vi "DeleteSearch.vi"(10 "EventQueue":T2(array[cluster]), 11 "Event":T3) -> (2 "Found":bool, 3 "Index":i32)   [LabVIEW 2014]
uses:
  TypeDefs/Point2D.ctl
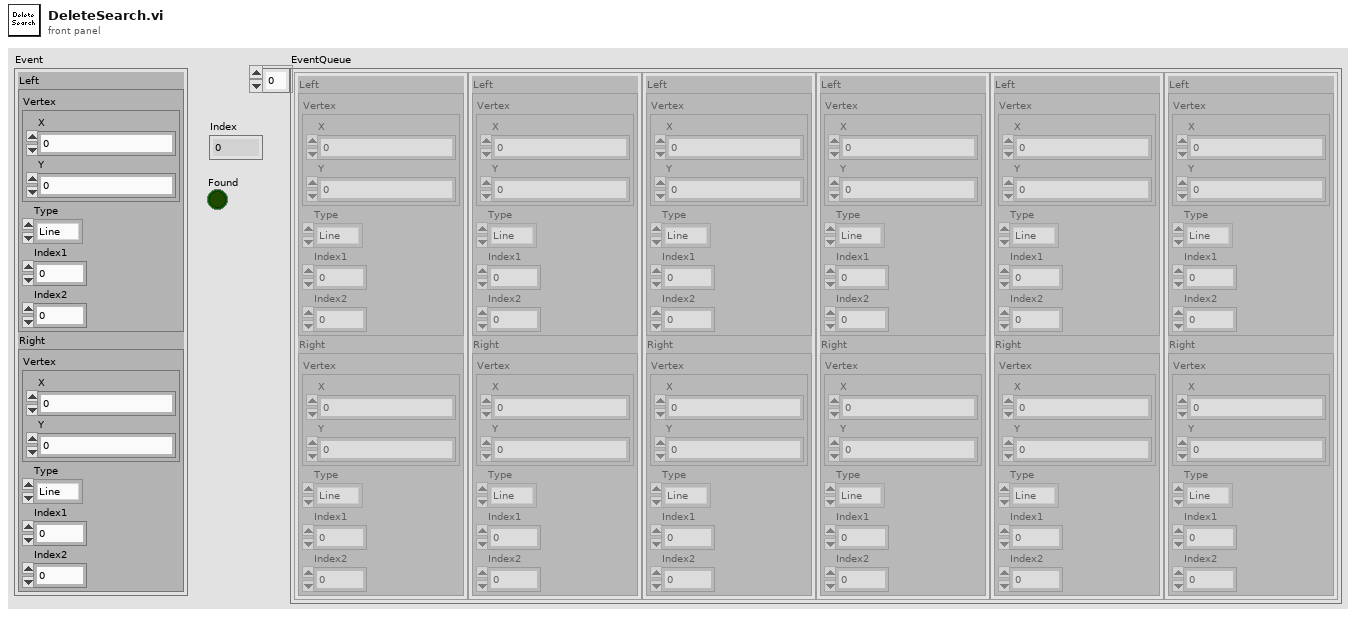
[diagram p1: front panel]
types:
  T1 = typedef "Point2D.ctl" = cluster{"X":sgl, "Y":sgl}
  T2 = cluster{"Left":cluster{"Vertex":T1, "Type":enum16{"Line", "Poly", "Cross"}, "Index1":i32, "Index2":i32}, "Right":cluster{"Vertex":T1, "Type":enum16{"Line", "Poly", "Cross"}, "Index1":i32, "Index2":i32}}[]
  T3 = cluster{"Left":cluster{"Vertex":T1, "Type":enum16{"Line", "Poly", "Cross"}, "Index1":i32, "Index2":i32}, "Right":cluster{"Vertex":T1, "Type":enum16{"Line", "Poly", "Cross"}, "Index1":i32, "Index2":i32}}
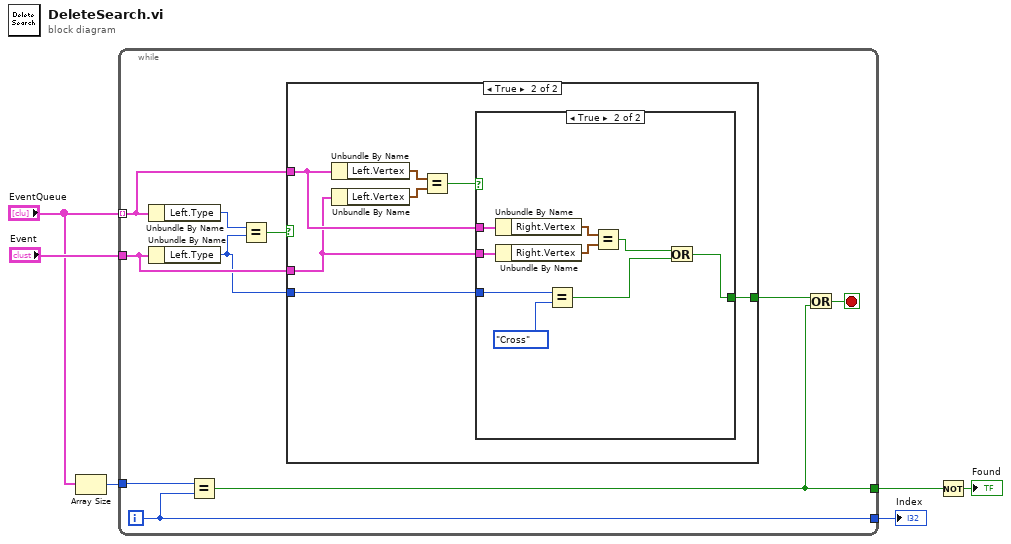
[diagram p0: block diagram]
diagram:
  n1 = Array Size(array="EventQueue") -> (size(s)=w3:i32)
  n2 = while {
    tunnel: "EventQueue" -> [w14] mode=indexing
    tunnel: "Event" -> [w13]
    tunnel: [w10] -> w5
    tunnel: w3 -> [w11]
    tunnel: [w7] -> w1
    i -> [w10]
    stop <- w8 stop-if-true
    n3 = Unbundle By Name(w14) -> ("Left.Type"=w16:enum16{"Line", "Poly", "Cross"})
    n4 = Unbundle By Name(w13) -> ("Left.Type"=w12:enum16{"Line", "Poly", "Cross"})
    n5 = Equal?(x=w11, y=w10) -> (x = y?=w7:bool)
    n6 = Equal?(x=w16, y=w12) -> (x = y?=w15:bool)
    n7 = case shown="True" w15 {
      tunnel: w14 -> [_ w20]
      tunnel: w13 -> [_ w19]
      tunnel: w12 -> [_ w18]
      tunnel: [_ w17] -> w9
      frame False {
      }
      frame True {
        n8 = Unbundle By Name(w20) -> ("Left.Vertex"=w23:T1)
        n9 = Unbundle By Name(w19) -> ("Left.Vertex"=w22:T1)
        n10 = Equal?(x=w23, y=w22) -> (x = y?=w21:bool)
        n11 = case shown="True" w21 {
          tunnel: w20 -> [_ w30]
          tunnel: w19 -> [_ w29]
          tunnel: w18 -> [_ w28]
          tunnel: [_ w24] -> w17
          frame False {
          }
          frame True {
            n12 = Unbundle By Name(w30) -> ("Right.Vertex"=w31:T1)
            n13 = Unbundle By Name(w29) -> ("Right.Vertex"=w32:T1)
            n14 = Equal?(x=w28, y=enum16{"Line", "Poly", "Cross"}."Cross") -> (x = y?=w25:bool)
            n15 = Equal?(x=w31, y=w32) -> (x = y?=w26:bool)
            n16 = Or(x=w26, y=w25) -> (x .or. y?=w24:bool)
          }
        }
      }
    }
    n17 = Or(x=w9, y=w7) -> (x .or. y?=w8:bool)
  }
  "Index" <- w5
  n18 = Not(x=w1) -> (.not. x?=→"Found":bool)
